vi "Receive Speeds.vi"() -> (1 "Fast":dbl, 2 "Slow":dbl, 3 "Tower":dbl)   [LabVIEW 2012]
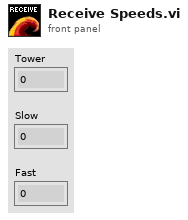
[diagram p1: front panel]
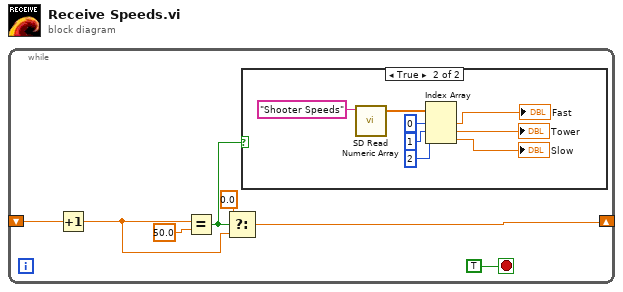
[diagram p0: block diagram]
diagram:
  n1 = while {
    shift-right: [w4] -> _
    shift-left: _ -> [w3]
    stop <- TRUE stop-if-true
    n2 = Increment(x=w3) -> (x+1=w2:dbl)
    n3 = Equal?(x=w2, y=50.0) -> (x = y?=w1:bool)
    n4 = Select(t=0.0, s=w1, f=w2) -> (s? t:f=w4:dbl)
    n5 = case shown="True" w1 {
      frame False {
      }
      frame True {
        n6 = call <vilib>:"SD Read Numeric Array.vi"("Name"="Shooter Speeds") -> ("Numeric Array"=w11:dbl[])  [unwired: 8 in, 2 out]
        n7 = Index Array(array=w11, index #1=0 ("index"), index #2=1 ("index"), index #3=2 ("index")) -> (element #1=→"Fast":dbl, element #2=→"Tower":dbl, element #3=→"Slow":dbl)
      }
    }
  }
